vi "双路单通通断器（U8[]）.vi"(7 "默认值":u8, 9 "X直通？":bool[](array[boolean]), 10 "Y_In":u8[](array[numeric]), 11 "X_In":u8[](array[numeric])) -> (2 "Y_Out":u8[](array[numeric]), 3 "X_Out":u8[](array[numeric]))   [LabVIEW 2011]
doc: "功能：\n\n返回一个枚举，表明输入数的范围，用于三段比较。\n\n\nCSXCS_366创建。"
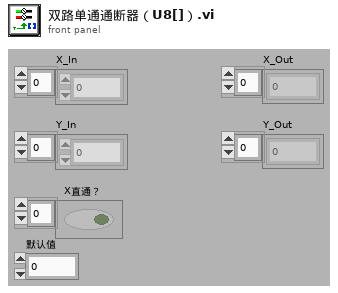
[diagram p1: front panel]
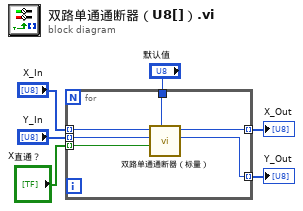
[diagram p0: block diagram]
diagram:
  n1 = for {
    tunnel: "X_In" -> [w12] mode=indexing
    tunnel: "Y_In" -> [w11] mode=indexing
    tunnel: "X直通？" -> [w10] mode=indexing
    tunnel: "默认值" -> [w9]
    tunnel: [w8] -> w2 mode=indexing
    tunnel: [w7] -> w1 mode=indexing
    n2 = call-poly "双路单通通断器（标量）.vi"("默认值"=w9, "X直通？"=w10, "Y_In"=w11, "X_In"=w12) -> ("Y_Out"=w7:u8, "X_Out"=w8:u8)  [unwired: 6 in]
  }
  "X_Out" <- w2
  "Y_Out" <- w1
